vi "Read Numeric Extensions.vi"(11 "Serializer.JSON in":refnum<class "Serializer.JSON.lvclass">) -> (2 "Numeric Extensions":bool, 3 "Serializer.JSON out":refnum<class "Serializer.JSON.lvclass">)   [LabVIEW 2013, in "OpenSerializer.JKI-JSON.lvlib" / "Serializer.JSON.lvclass"]
uses:
  Serializer.JSON.lvclass
  Serializer.JSON.lvclass/Serializer.JSON.ctl
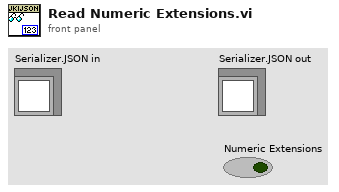
[diagram p1: front panel]
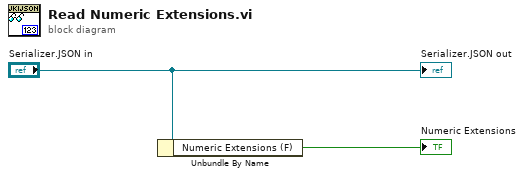
[diagram p0: block diagram]
diagram:
  n1 = Unbundle By Name("Serializer.JSON in") -> ("Numeric Extensions (F)"=→"Numeric Extensions":bool)
  "Serializer.JSON out" <- "Serializer.JSON in"
